vi "ForwardForInch.vi"(10 "Distance":dbl, 11 "RobotDriveDevRef":T1={"DevStatus"={"status"=FALSE, "code"=0, "source"=""}, "Motors[]"=[], "Square Inputs"=FALSE, "Max Output"=1.0}) -> (3 "RobotDriveDevRef 2":T1={"DevStatus"={"status"=FALSE, "code"=0, "source"=""}, "Motors[]"=[], "Square Inputs"=FALSE, "Max Output"=1.0})   [LabVIEW 2016]
uses:
  <vilib>/Rock Robotics/WPI/RobotDrive/WPI_RobotDriveDevRef.ctl
  <vilib>/Rock Robotics/WPI/MotorControl/WPI_MotorControlDeviceRef.ctl
  <vilib>/Rock Robotics/WPI/MotorControl/WPI_MotorControlType.ctl
  <vilib>/Rock Robotics/SystemInterfaces/DIO/FPGA_DIOPWMChannel.ctl
  <vilib>/Rock Robotics/WPI/PWM/WPI_PWMDeadband.ctl
  <vilib>/Rock Robotics/WPI/RobotDrive/WPI_RobotDriveArcadeDrive_Standard(NoSaturation).vi
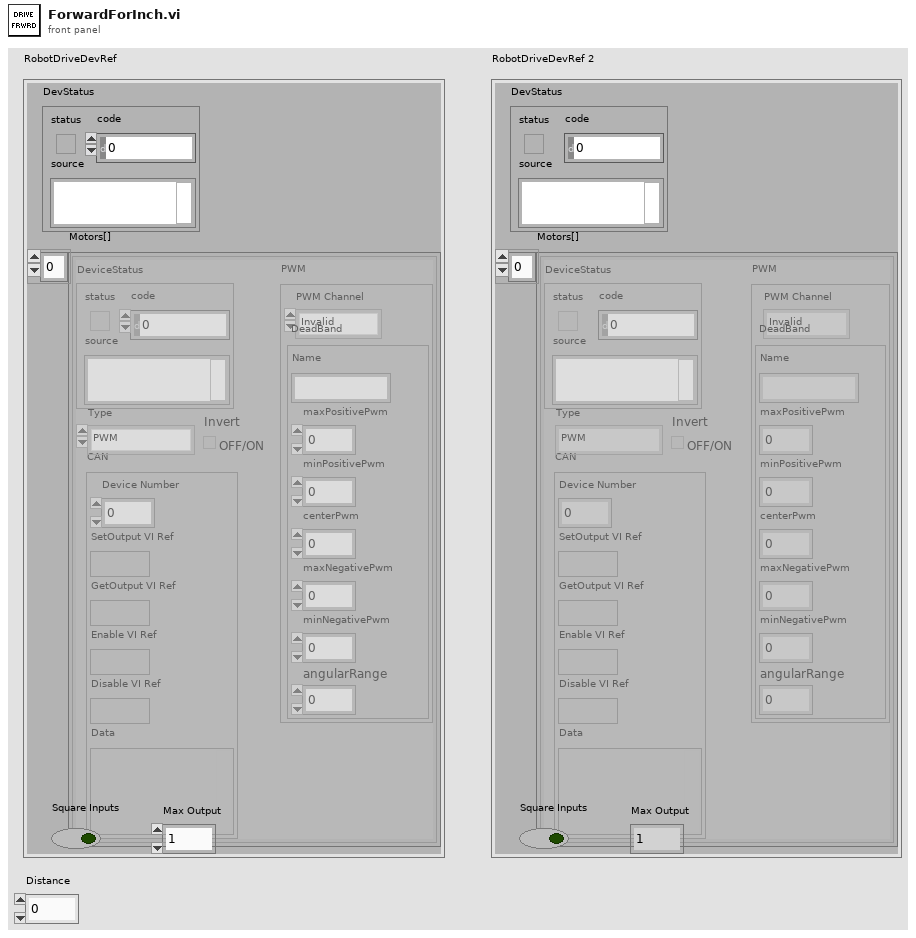
[diagram p1: front panel]
types:
  T1 = typedef "WPI_RobotDriveDevRef.ctl" = cluster{"DevStatus":errorcluster, "Motors[]":T2[], "Square Inputs":bool, "Max Output":dbl}
  T2 = typedef "WPI_MotorControlDeviceRef.ctl" = cluster{"DeviceStatus":errorcluster, "Type":T3, "PWM":cluster{"PWM Channel":T4, "DeadBand":T5}, "CAN":cluster{"Device Number":u8, "SetOutput VI Ref":variant, "GetOutput VI Ref":variant, "Enable VI Ref":variant, "Disable VI Ref":variant, "Data":variant}, "Invert":bool}
  T3 = typedef "WPI_MotorControlType.ctl" = enum16{"PWM", "CAN"}
  T4 = typedef "FPGA_DIOPWMChannel.ctl" = enum8{"PWM 0", "PWM 1", "PWM 2", "PWM 3", "PWM 4", "PWM 5", "PWM 6", "PWM 7", "PWM 8", "PWM 9", "PWM MXP 0", "PWM MXP 1", "PWM MXP 2", "PWM MXP 3", "PWM MXP 4", "PWM MXP 5", "PWM MXP 6", "PWM MXP 7", "PWM MXP 8", "PWM MXP 9", "Invalid"}
  T5 = typedef "WPI_PWMDeadband.ctl" = cluster{"Name":string, "maxPositivePwm":i32, "minPositivePwm":i32, "centerPwm":i32, "maxNegativePwm":i32, "minNegativePwm":i32, "angularRange":u16}
  T6 = typedef "WPI_EncoderDevRef.ctl" = cluster{"DevStatus":errorcluster, "EncoderIndex":T7, "CounterIndex":T8, "DistancePerCount":dbl, "Decoding Type":T9}
  T7 = typedef "FPGA_EncoderIdx.ctl" = enum8{"Enc 0", "Enc 1", "Enc 2", "Enc 3", "Enc 4", "Enc 5", "Enc 6", "Enc 7", "Invalid"}
  T8 = typedef "FPGA_CounterCtrSystemIndex.ctl" = enum8{"Ctr 0", "Ctr 1", "Ctr 2", "Ctr 3", "Ctr 4", "Ctr 5", "Ctr 6", "Ctr 7", "Invalid"}
  T9 = typedef "WPI_EncoderType.ctl" = enum16{"1x", "2x", "4x"}
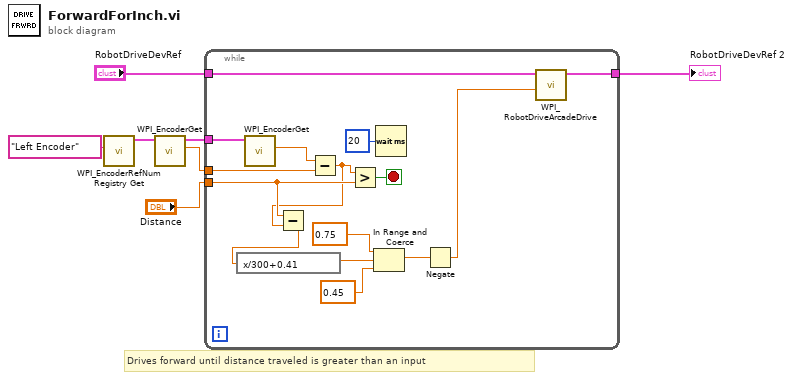
[diagram p0: block diagram]
diagram:
  # "Drives forward until distance traveled is greater than an input"
  n1 = call <vilib>:"WPI_EncoderRefNum Registry Get.vi"("refnum name"="Left Encoder") -> ("EncoderDevRef"=w6:T6)  [unwired: 9 in, 1 out]
  n2 = call <vilib>:"WPI_EncoderGet.vi"("EncoderDevRef"=w6) -> ("Distance"=w5:dbl, "EncoderDevRef"=w4:T6)  [unwired: 5 in, 4 out]
  n3 = while {
    tunnel: w5 -> [w20]
    tunnel: w4 -> [w22]
    tunnel: "Distance" -> [w10]
    tunnel: "RobotDriveDevRef" -> [w18]
    tunnel: [w17] -> w1
    stop <- w19 stop-if-true
    n4 = call <vilib>:"WPI_EncoderGet.vi"("EncoderDevRef"=w22) -> ("Distance"=w21:dbl)  [unwired: 5 in, 5 out]
    n5 = Subtract(x=w21, y=w20) -> (x-y=w9:dbl)
    n6 = Subtract(x=w10, y=w9) -> (x-y=w8:dbl)
    n7 = expression code="x/300+0.41"(w8) -> (w12:dbl)
    n8 = Greater?(x=w9, y=w10) -> (0:w19:bool)
    n9 = In Range and Coerce(upper limit=0.75, x=w12, lower limit=0.45) -> (coerced(x)=w15:dbl)  [unwired: 1 out]
    n10 = Wait (ms)(milliseconds to wait=u32 20) -> ()  [unwired: 1 out]
    n11 = Negate(x=w15) -> (-x=w11:dbl)
    n12 = call-poly <vilib>:"WPI_RobotDriveArcadeDrive.vi"("Y axis value"=w11, "RobotDriveDevRef"=w18) -> ("RobotDriveDevRef"=w17:T1)  [unwired: 7 in, 2 out]
  }
  "RobotDriveDevRef 2" <- w1
